vi "PmodALSOpen.vi"(7 "SPI Channel (0)":u8, 8 "error in (no error)":errorcluster, 11 "LINX Ref":T1) -> (0 "error out":errorcluster, 2 "Actual Clock Frequency":u32, 3 "LINX Resource":T1)   [LabVIEW 2014]
doc: "Open a connection to the PmodALS.\n\nConfigure the specified SPI channel.\n\nClock Frequency: Specify the desired SPI clock frequency. The default clock frequency for the PmodALS is between 1 and 4MHz. 4MHz is the default value.\n\nThis VI outputs the actual achieved clock frequency.\n\nBit Order: Specify the order in which bits are shifted out. PmodALS is MSb first.\n\nSPI Mode: Chose the SPI mode to determine the clock idle value and sampling edge. PmodALS is Mode 0 (clock idle low; data sampled on rising edge)."
uses:
  <vilib>/MakerHub/LINX/Private/Type Defs/LINX Ref.ctl
  <vilib>/MakerHub/LINX/Private/Type Defs/Platform.ctl
  <vilib>/MakerHub/LINX/Private/Type Defs/Interface.ctl
  <vilib>/MakerHub/LINX/Private/Device/Type Defs/LINX Device Config.ctl
  <vilib>/MakerHub/LINX/Private/Device/Type Defs/TCP Config.ctl
  <vilib>/MakerHub/LINX/Private/Device/Type Defs/Channels.ctl
  <vilib>/MakerHub/LINX/Private/Type Defs/Peripherals/SPI/SPI Configuration.ctl
  <vilib>/MakerHub/LINX/Private/Type Defs/Peripherals/SPI/SPI Bit Order.ctl
  <vilib>/MakerHub/LINX/Private/Type Defs/Peripherals/SPI/SPI Mode.ctl
  <vilib>/MakerHub/LINX/LMH-LINX.lvlib
  <vilib>/MakerHub/LINX/Private/Device/Device.lvlib
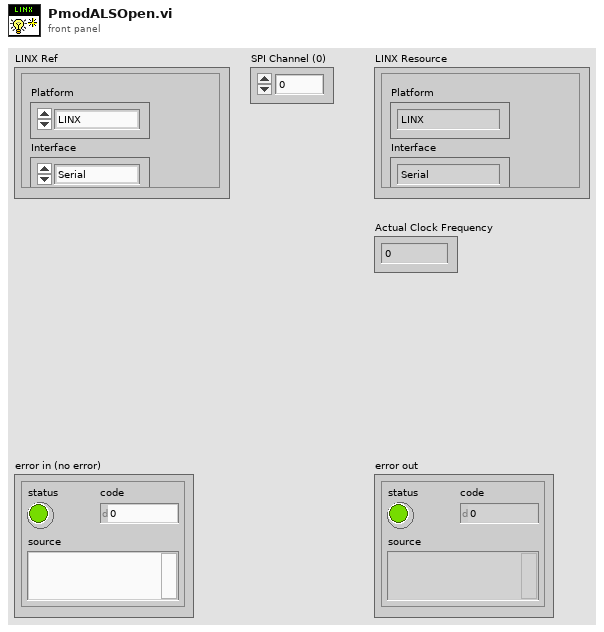
[diagram p1: front panel]
types:
  T1 = typedef "LMH-LINX.lvlib/LINX Ref.ctl" = cluster{"Platform":T2, "Interface":T3, "LINX Device Config":T4}
  T2 = typedef "LMH-LINX.lvlib/Platform.ctl" = enum16{"LINX", "myRIO"}
  T3 = typedef "LMH-LINX.lvlib/Interface.ctl" = enum16{"Serial", "TCP"}
  T4 = typedef "LMH-LINX.lvlib/Device.lvlib/LINX Device Config.ctl" = cluster{"Interface":T3, "COM Port":refnum<visa-resource-name>, "TCP Configuration":T5, "Device Family":u8, "Device ID":u8, "Device Name":string, "TCP Ref":refnum<k5>, "Channels":T6}
  T5 = typedef "LMH-LINX.lvlib/Device.lvlib/TCP Config.ctl" = cluster{"IP Address":string, "Port":u16}
  T6 = typedef "LMH-LINX.lvlib/Channels.ctl" = cluster{"DI":u8[], "DO":u8[], "AI":u8[], "AO":u8[], "PWM":u8[], "QE":u8[], "UART":u8[], "I2C 2":u8[], "SPI":u8[], "CAN":u8[], "Servo":u8[], "AI Ref (V)":dbl, "AO Ref (V)":dbl, "AO Resolution (Bits)":u8}
  T7 = typedef "LMH-LINX.lvlib/SPI Configuration.ctl" = cluster{"Clock Frequency":u32, "Bit Order":T8, "SPI Mode":T9}
  T8 = typedef "LMH-LINX.lvlib/SPI Bit Order.ctl" = enum8{"LSb First", "MSb First"}
  T9 = typedef "LMH-LINX.lvlib/SPI Mode.ctl" = enum8{"Mode 0", "Mode 1", "Mode 2", "Mode 3"}
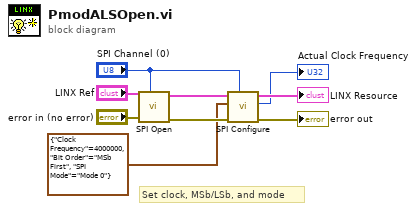
[diagram p0: block diagram]
diagram:
  # "Set clock, MSb/LSb, and mode"
  n1 = call <vilib>:"SPI Open.vi"("SPI Channel (0)"="SPI Channel (0)", "Error In"="error in (no error)", "LINX Resource"="LINX Ref") -> ("Error Out"=w5:errorcluster, "LINX Resource"=w4:T1)  [unwired: 7 in]
  n2 = call <vilib>:"SPI Configure.vi"("SPI Channel (0)"="SPI Channel (0)", "Error In"=w5, "SPI Configuration"=T7 {"Clock Frequency"=4000000, "Bit Order"=enum."MSb First", "SPI Mode"=enum."Mode 0"}, "LINX Resource"=w4) -> ("Error Out"=→"error out":errorcluster, "Actual Clock Frequency"=→"Actual Clock Frequency":u32, "LINX Resource"=→"LINX Resource":T1)  [unwired: 5 in]
